vi "ch_switch.vi"(0 "channel 14":bool, 1 "channel 4":bool, 2 "channel 13":bool, 3 "channel 5":bool, 4 "channel 12":bool, 5 "channel 6":bool, 6 "channel 7":bool, 8 "channel 3":bool, 9 "channel 8":bool, 10 "channel 15":bool, 11 "channel 9":bool, 12 "channel 2":bool, 13 "channel 10":bool, 14 "channel 1":bool, 15 "channel 11":bool, 16 "channel 0":bool, 18 "Array in":dbl[](array[numeric])) -> (20 "Array out":dbl[](array[numeric]))   [LabVIEW 2020]
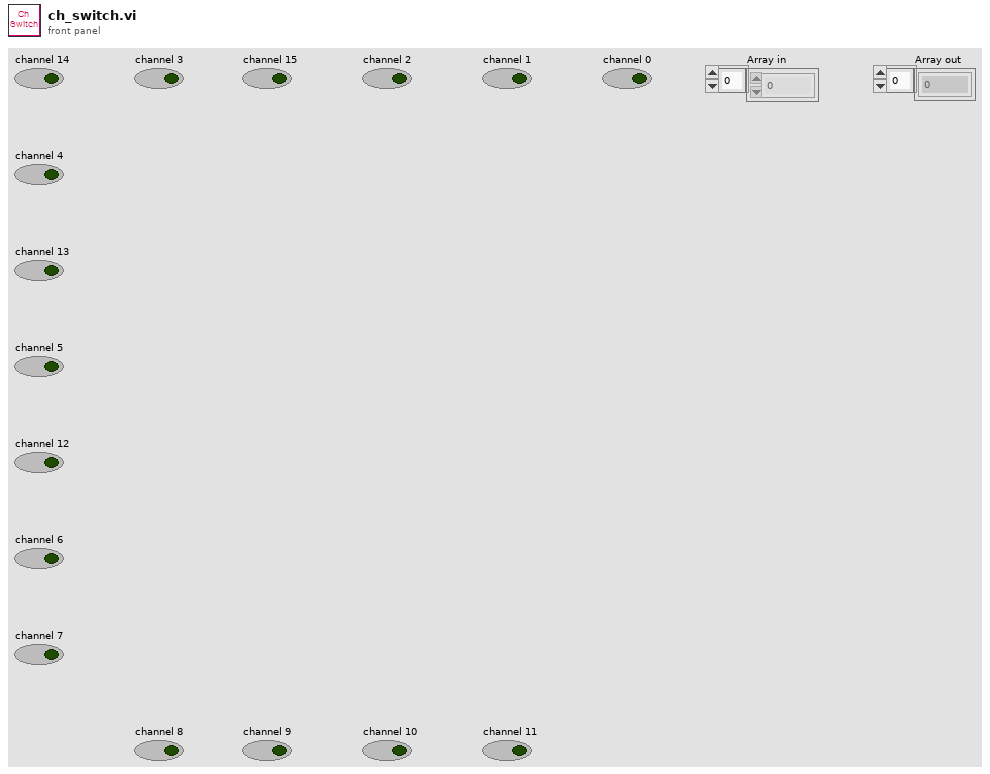
[diagram p1: front panel]
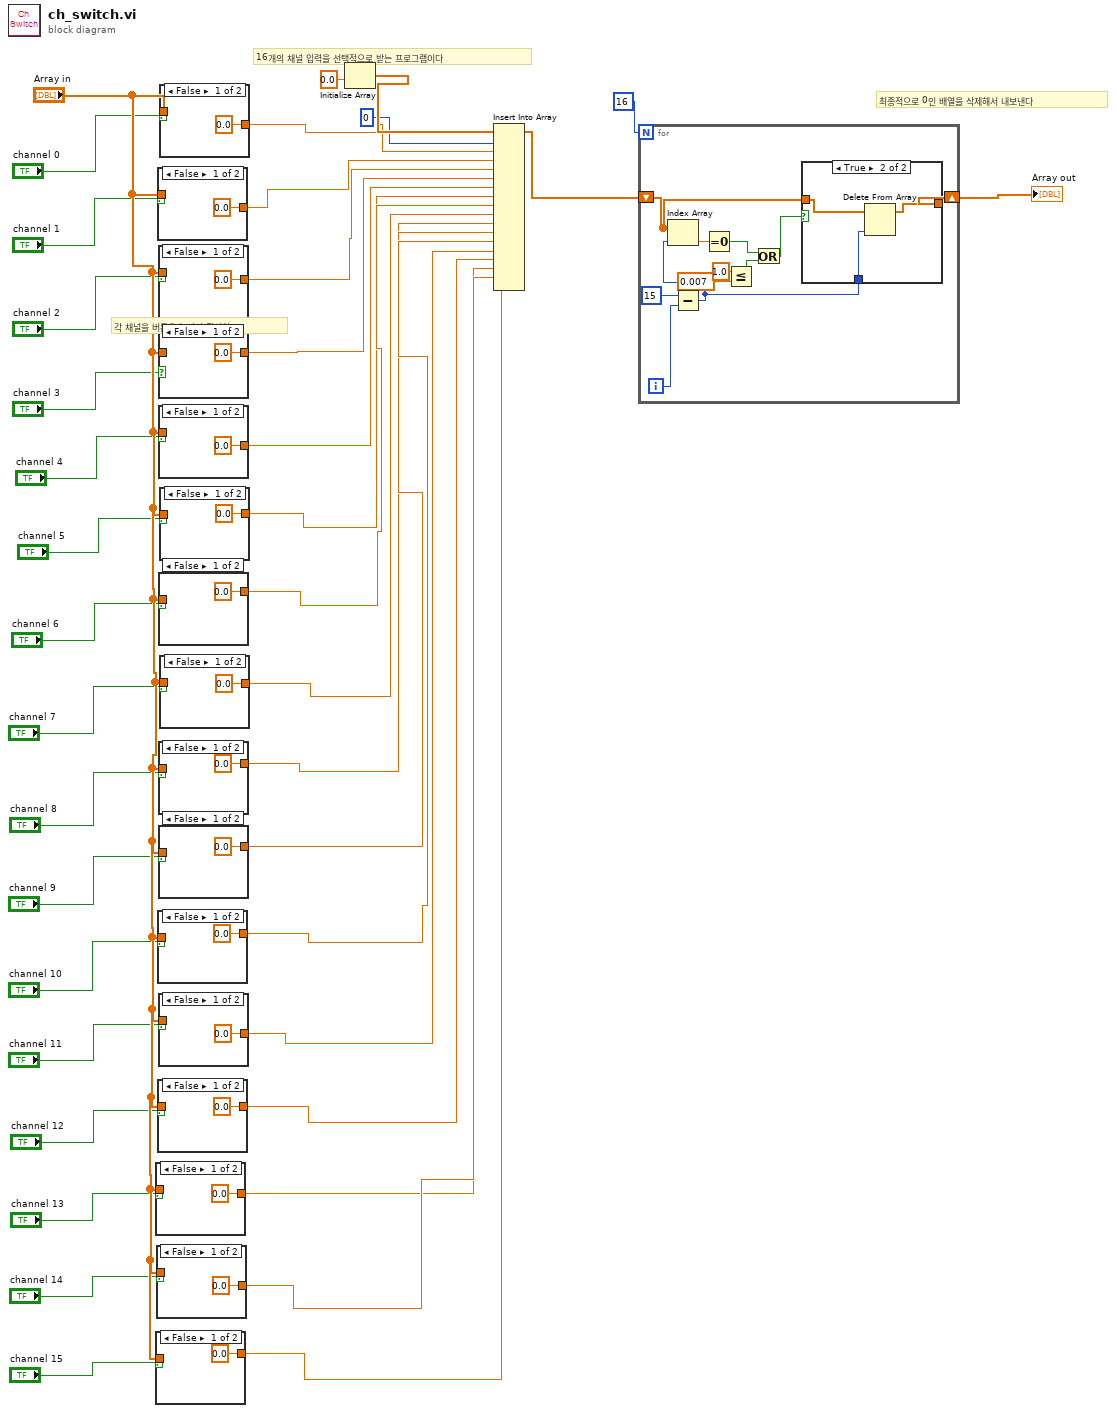
[diagram p0: block diagram]
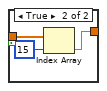
[diagram p3: hidden frame]
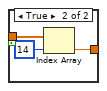
[diagram p4: hidden frame]
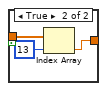
[diagram p5: hidden frame]
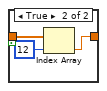
[diagram p6: hidden frame]
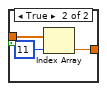
[diagram p7: hidden frame]
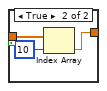
[diagram p8: hidden frame]
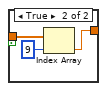
[diagram p9: hidden frame]
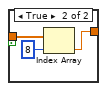
[diagram p10: hidden frame]
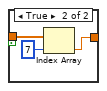
[diagram p11: hidden frame]
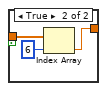
[diagram p12: hidden frame]
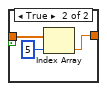
[diagram p13: hidden frame]
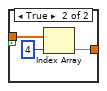
[diagram p14: hidden frame]
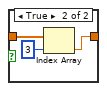
[diagram p15: hidden frame]
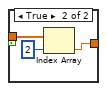
[diagram p16: hidden frame]
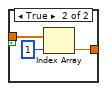
[diagram p17: hidden frame]
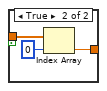
[diagram p18: hidden frame]
diagram:
  # "최종적으로 0인 배열을 삭제해서 내보낸다"
  # "각 채널을 버튼을 눌러서 활성화"
  # "16개의 채널 입력을 선택적으로 받는 프로그램이다"
  n1 = case shown="False" "channel 13" {
    tunnel: "Array in" -> [_ w42]
    tunnel: [0.0 ("element") w41] -> w34
    frame False {
    }
    frame True {
      n2 = Index Array(array=w42, index=13) -> (element=w41:dbl)
    }
  }
  n3 = case shown="False" "channel 15" {
    tunnel: "Array in" -> [_ w46]
    tunnel: [0.0 ("element") w45] -> w36
    frame False {
    }
    frame True {
      n4 = Index Array(array=w46, index=15) -> (element=w45:dbl)
    }
  }
  n5 = case shown="False" "channel 14" {
    tunnel: "Array in" -> [_ w50]
    tunnel: [0.0 ("element") w49] -> w35
    frame False {
    }
    frame True {
      n6 = Index Array(array=w50, index=14) -> (element=w49:dbl)
    }
  }
  n7 = case shown="False" "channel 1" {
    tunnel: "Array in" -> [_ w54]
    tunnel: [0.0 ("element") w53] -> w22
    frame False {
    }
    frame True {
      n8 = Index Array(array=w54, index=1) -> (element=w53:dbl)
    }
  }
  n9 = case shown="False" "channel 10" {
    tunnel: "Array in" -> [_ w58]
    tunnel: [0.0 ("element") w57] -> w31
    frame False {
    }
    frame True {
      n10 = Index Array(array=w58, index=10) -> (element=w57:dbl)
    }
  }
  n11 = case shown="False" "channel 12" {
    tunnel: "Array in" -> [_ w62]
    tunnel: [0.0 ("element") w61] -> w33
    frame False {
    }
    frame True {
      n12 = Index Array(array=w62, index=12) -> (element=w61:dbl)
    }
  }
  n13 = case shown="False" "channel 2" {
    tunnel: "Array in" -> [_ w66]
    tunnel: [0.0 ("element") w65] -> w23
    frame False {
    }
    frame True {
      n14 = Index Array(array=w66, index=2) -> (element=w65:dbl)
    }
  }
  n15 = case shown="False" "channel 3" {
    tunnel: "Array in" -> [_ w70]
    tunnel: [0.0 ("element") w69] -> w24
    frame False {
    }
    frame True {
      n16 = Index Array(array=w70, index=3) -> (element=w69:dbl)
    }
  }
  n17 = case shown="False" "channel 4" {
    tunnel: "Array in" -> [_ w74]
    tunnel: [0.0 ("element") w73] -> w25
    frame False {
    }
    frame True {
      n18 = Index Array(array=w74, index=4) -> (element=w73:dbl)
    }
  }
  n19 = case shown="False" "channel 6" {
    tunnel: "Array in" -> [_ w78]
    tunnel: [0.0 ("element") w77] -> w27
    frame False {
    }
    frame True {
      n20 = Index Array(array=w78, index=6) -> (element=w77:dbl)
    }
  }
  n21 = case shown="False" "channel 8" {
    tunnel: "Array in" -> [_ w82]
    tunnel: [0.0 ("element") w81] -> w29
    frame False {
    }
    frame True {
      n22 = Index Array(array=w82, index=8) -> (element=w81:dbl)
    }
  }
  n23 = case shown="False" "channel 9" {
    tunnel: "Array in" -> [_ w86]
    tunnel: [0.0 ("element") w85] -> w30
    frame False {
    }
    frame True {
      n24 = Index Array(array=w86, index=9) -> (element=w85:dbl)
    }
  }
  n25 = case shown="False" "channel 11" {
    tunnel: "Array in" -> [_ w90]
    tunnel: [0.0 ("element") w89] -> w32
    frame False {
    }
    frame True {
      n26 = Index Array(array=w90, index=11) -> (element=w89:dbl)
    }
  }
  n27 = case shown="False" "channel 0" {
    tunnel: "Array in" -> [_ w94]
    tunnel: [0.0 ("element") w93] -> w20
    frame False {
    }
    frame True {
      n28 = Index Array(array=w94, index=0) -> (element=w93:dbl)
    }
  }
  n29 = case shown="False" "channel 5" {
    tunnel: "Array in" -> [_ w98]
    tunnel: [0.0 ("element") w97] -> w26
    frame False {
    }
    frame True {
      n30 = Index Array(array=w98, index=5) -> (element=w97:dbl)
    }
  }
  n31 = case shown="False" "channel 7" {
    tunnel: "Array in" -> [_ w102]
    tunnel: [0.0 ("element") w101] -> w28
    frame False {
    }
    frame True {
      n32 = Index Array(array=w102, index=7) -> (element=w101:dbl)
    }
  }
  n33 = Initialize Array(0.0 ("element")) -> (w21:dbl[])  [unwired: 1 in]
  n34 = Insert Into Array(array=w21, index=0, new element #1=w20, new element #2=w22, new element #3=w23, new element #4=w24, new element #5=w25, new element #6=w26, new element #7=w27, new element #8=w28, new element #9=w29, new element #10=w30, new element #11=w31, new element #12=w32, new element #13=w33, new element #14=w34, new element #15=w35, new element #16=w36) -> (w38:dbl[])
  n35 = for {
    N: 16 -> [_]
    shift-right: [w110] -> w39
    shift-left: w38 -> [w111]
    i -> [w114]
    n36 = Subtract(x=15, y=w114) -> (x-y=w112:i32)
    n37 = Index Array(array=w111, index=w112) -> (element=w105:dbl)
    n38 = Equal To 0?(x=w105) -> (x = 0?=w109:bool)
    n39 = Less Or Equal?(x=1.0, y=0.007) -> (x <= y?=w107:bool)
    n40 = Or(x=w109, y=w107) -> (x .or. y?=w108:bool)
    n41 = case shown="True" w108 {
      tunnel: w112 -> [_ w118]
      tunnel: w111 -> [w115 w117]
      tunnel: [w115 w116] -> w110
      frame False {
      }
      frame True {
        n42 = Delete From Array(array=w117, index=w118) -> (array with subset deleted=w116:dbl[])  [unwired: 1 in, 1 out]
      }
    }
  }
  "Array out" <- w39
